vi "Calclengthes.vi"(6 "error in (no error)":errorcluster, 8 "DutyCluster":T1 {"Iteration" items=["first iteration", "second iteration"]}, 9 "XYZ coordinates (um)":dbl[][](array[numeric])) -> (0 "error out":errorcluster, 3 "difference":dbl[](array[numeric]))   [LabVIEW 2010]
uses:
  TypeDefs/DutyCluster.ctl
  <vilib>/Analysis/NI_AALPro.lvlib
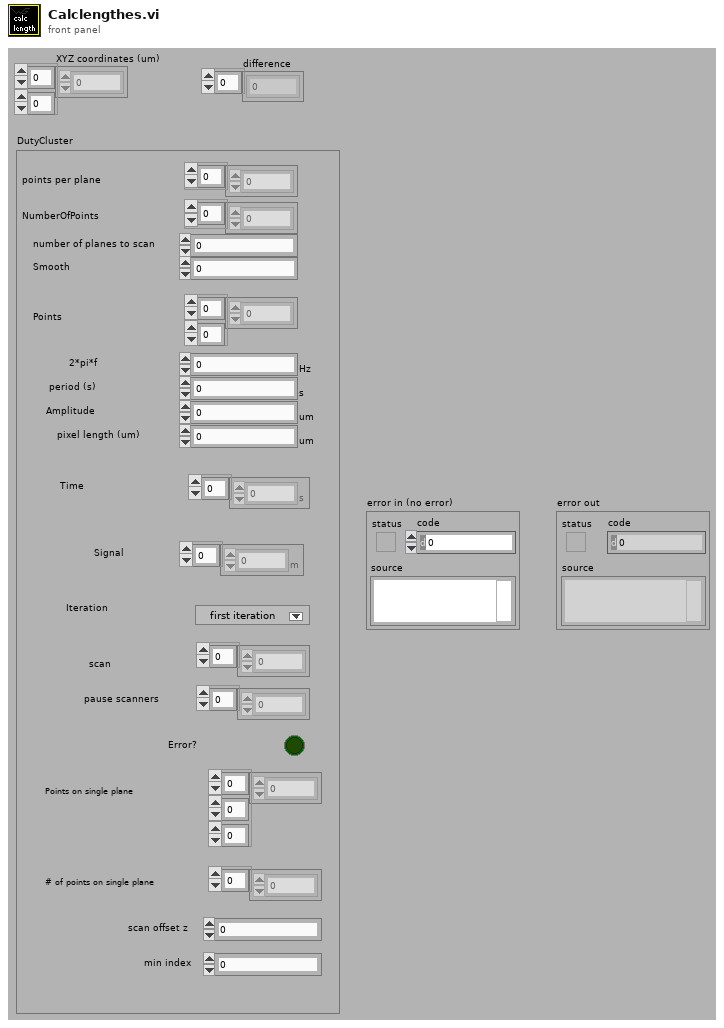
[diagram p1: front panel]
types:
  T1 = typedef "DutyCluster.ctl" = cluster{"points per plane":i32[], "NumberOfPoints":i32[], "number of planes to scan":i32, "Smooth":i32, "Points":dbl[][], "2*pi*f":dbl[unit], "period (s)":dbl[unit], "Amplitude":dbl[unit], "pixel length (um)":dbl[unit], "Time":dbl[unit][], "Signal":dbl[unit][], "Iteration":u16, "scan":i32[], "pause scanners":i32[], "Error?":bool, "Points on single plane":dbl[][][], "# of points on single plane":i32[], "scan offset z":i32, "min index":i32}
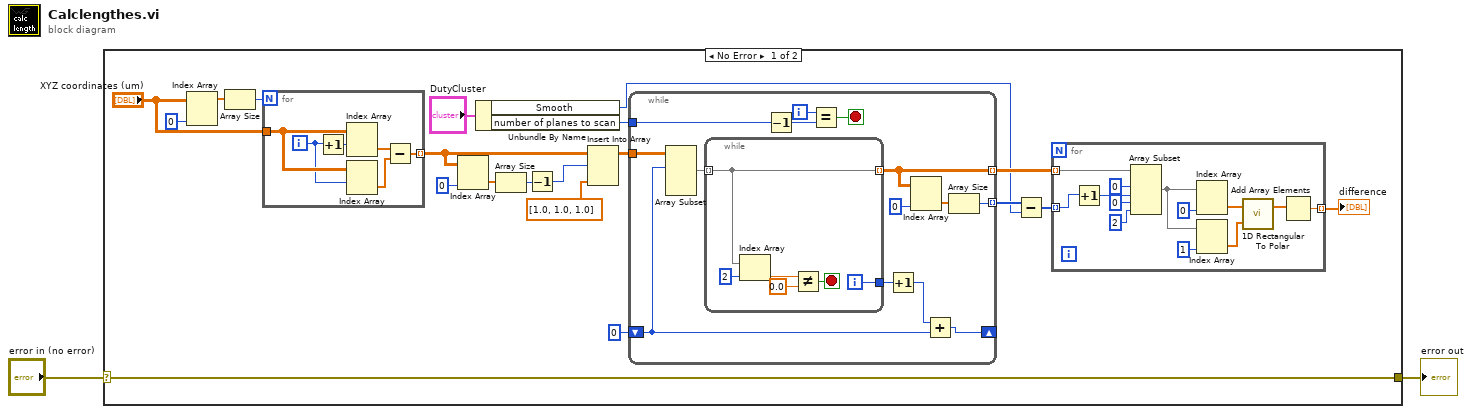
[diagram p0: block diagram]
diagram:
  n1 = case shown="No Error" "error in (no error)" {
    selector: "error in (no error)" -> [w3 w62]
    tunnel: [w3 w62] -> w1
    frame No Error {
      n2 = Index Array(array="XYZ coordinates (um)", index (col)=0 ("disabled index (col)")) -> (element=w21:dbl[])  [unwired: 1 in]
      n3 = Array Size(array=w21) -> (size(s)=w20:i32)
      n4 = for {
        N: w20 -> [_]
        tunnel: "XYZ coordinates (um)" -> [w61]
        tunnel: [w56] -> w16 mode=indexing
        i -> [w59]
        n5 = Increment(x=w59) -> (x+1=w60:i32)
        n6 = Index Array(array=w61, index (row)=w60) -> (element=w58:dbl[])  [unwired: 1 in]
        n7 = Index Array(array=w61, index (row)=w59) -> (element=w57:dbl[])  [unwired: 1 in]
        n8 = Subtract(x=w58, y=w57) -> (x-y=w56:dbl[])
      }
      n9 = Index Array(array=w16, index (col)=0 ("disabled index (col)")) -> (element=w15:dbl[])  [unwired: 1 in]
      n10 = Unbundle By Name("DutyCluster") -> ("Smooth"=w4:i32, "number of planes to scan"=w5:i32)
      n11 = Array Size(array=w15) -> (size(s)=w13:i32)
      n12 = Decrement(x=w13) -> (x-1=w12:i32)
      n13 = Insert Into Array(array=w16, index (row)=w12, new element=dbl[] [1.0, 1.0, 1.0] ("new element/subarray")) -> (w14:dbl[][])  [unwired: 1 in]
      n14 = while {
        tunnel: w14 -> [w47]
        shift-right: [w49] -> _
        shift-left: 0 -> [w37]
        tunnel: [w40] -> w10 mode=indexing
        tunnel: [w39] -> w8 mode=indexing
        tunnel: w5 -> [w36]
        i -> [w46]
        stop <- w45 stop-if-true
        n15 = Array Subset(array=w47, index (row)=w37) -> (w48:dbl[][])  [unwired: 3 in]
        n16 = while {
          tunnel: w48 -> [w51] mode=indexing
          tunnel: [w51] -> w40 mode=indexing
          tunnel: [w50] -> w44
          i -> [w50]
          stop <- w52 stop-if-true
          n17 = Index Array(array=w51, index=2) -> (element=w53:dbl)
          n18 = Not Equal?(x=w53, y=0.0) -> (x != y?=w52:bool)
        }
        n19 = Decrement(x=w36) -> (x-1=w43:i32)
        n20 = Equal?(x=w46, y=w43) -> (x = y?=w45:bool)
        n21 = Increment(x=w44) -> (x+1=w38:i32)
        n22 = Index Array(array=w40, index (col)=0 ("disabled index (col)")) -> (element=w42:dbl[])  [unwired: 1 in]
        n23 = Add(x=w38, y=w37) -> (x+y=w49:i32)
        n24 = Array Size(array=w42) -> (size(s)=w39:i32)
      }
      n25 = Subtract(x=w8, y=w4) -> (x-y=w7:i32[])
      n26 = for {
        tunnel: w10 -> [w35] mode=indexing
        tunnel: [w26] -> w9 mode=indexing
        tunnel: w7 -> [w24] mode=indexing
        n27 = Increment(x=w24) -> (x+1=w23:i32)
        n28 = Array Subset(array=w35, index (row)=0 ("index"), length (row)=w23, index (col)=0 ("index"), length (col)=2 ("length")) -> (w27:dbl[][])
        n29 = Index Array(array=w27, index (col)=0 ("index")) -> (element=w32:dbl[])  [unwired: 1 in]
        n30 = Index Array(array=w27, index (col)=1 ("length")) -> (element=w31:dbl[])  [unwired: 1 in]
        n31 = call <vilib>:"1D Rectangular To Polar.vi"("X"=w32, "Y"=w31) -> ("Magnitude"=w30:dbl[])  [unwired: 2 out]
        n32 = Add Array Elements(numeric array=w30) -> (sum=w26:dbl)
      }
      "difference" <- w9
    }
    frame Error {
    }
  }
  "error out" <- w1
